vi "Relative Standard Deviation for two dimensional array.vi"(10 "Array - Numeric":dbl[][](array[numeric])) -> (0 "Min Value":dbl, 1 "Max Value":dbl, 2 "mean":dbl format="%0.2f", 3 "Relative Standard Deviation":dbl)   [LabVIEW 2016]
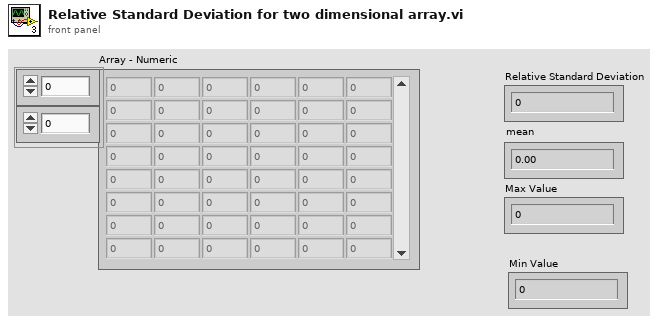
[diagram p1: front panel]
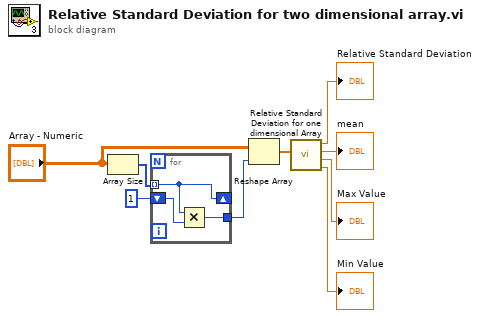
[diagram p0: block diagram]
diagram:
  n1 = Array Size(array="Array - Numeric") -> (size(s)=w9:i32[])
  n2 = for {
    tunnel: w9 -> [w11] mode=indexing
    shift-right: [w11] -> _
    shift-left: 1 -> [w12]
    tunnel: [w10] -> w6
    n3 = Multiply(x=w11, y=w12) -> (x*y=w10:i32)
  }
  n4 = Reshape Array("Array - Numeric", w6) -> (w5:dbl[])
  n5 = call "Relative Standard Deviation for one dimensional Array.vi"("Input Array"=w5) -> ("Min Value"=→"Min Value":dbl, "Max Value"=→"Max Value":dbl, "mean"=→"mean":dbl, "Relative Standard Deviation"=→"Relative Standard Deviation":dbl)  [unwired: 7 in]
